vi "email.vi"(1 "Body":string="[No Body]", 2 "Enable":bool) -> ()   [LabVIEW 2011]
panel:
  in  "CC (Carbon Copy Recipient - Optional) 2":string
  out "error out":errorcluster
  in  "CC (Carbon Copy Recipient - Optional)":string
  in  "Attachment - Optional":path
  in  "Port":i32=587
  in  "Enable SSL":bool=TRUE
  in  "GMAIL Account Password":string="joblhzitaafwukgr"
  in  "GMAIL Account User ID":string="hvac.labview"
  in  "Outgoing Mail Server (SMTP)":string="smtp.gmail.com"
  in  "Subject":string="Automatic Email: HVAC Project"
  in  "Recipient's Name":string="HVAC Member"
  in  "Recipient's Email":string="kth.ee.hvac@gmail.com"
  in  "Sender's Name":string="hvac.labview"
  in  "Sender's Email":string="hvac.labview@gmail.com"
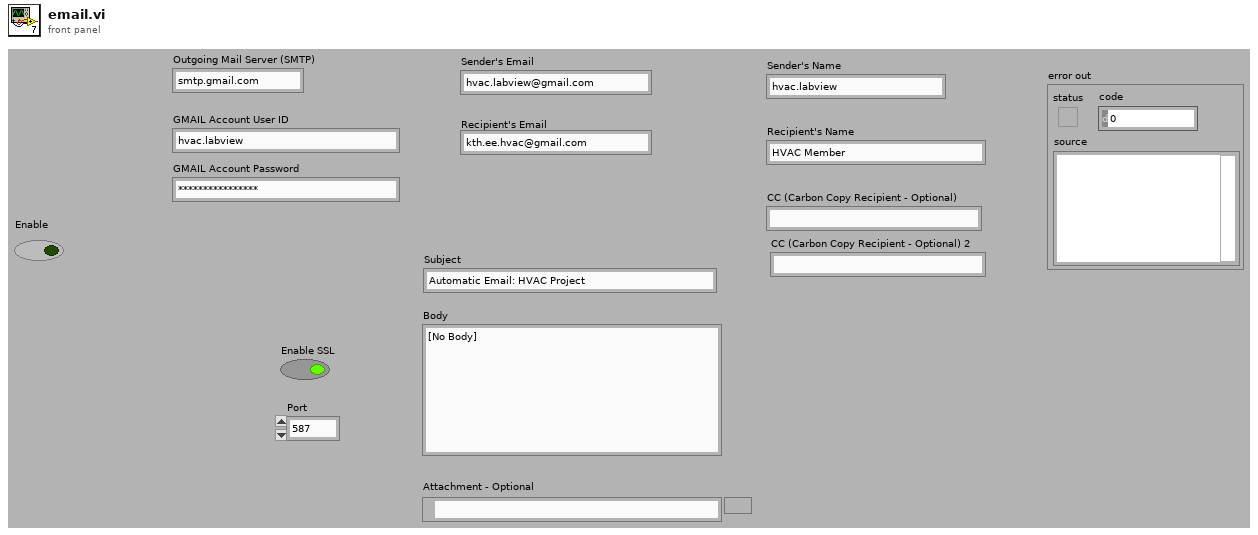
[diagram p1: front panel]
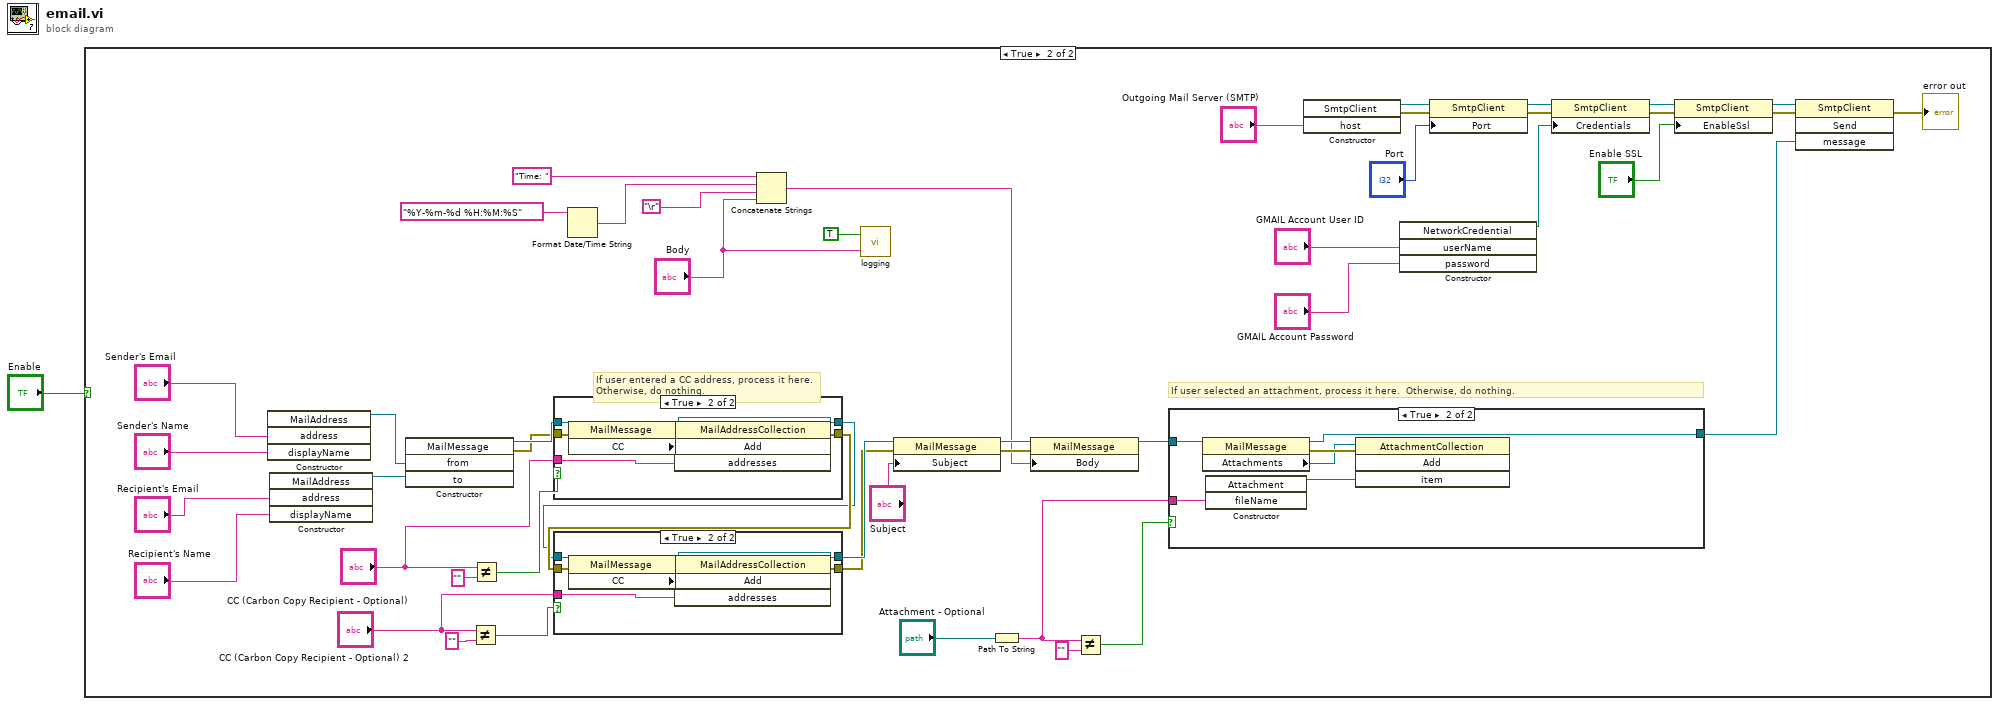
[diagram p0: block diagram]
diagram:
  n1 = case shown="True" "Enable" {
    frame False {
    }
    frame True {
      # "If user selected an attachment, process it here.  Otherwise, do nothing."
      # "If user entered a CC address, process it here.\nOtherwise, do nothing."
      n2 = constructor class="MailAddress"("address"="Sender's Email", "displayName"="Sender's Name") -> (reference out=w49:refnum<k24>)  [unwired: 3 in, 4 out]
      n3 = constructor class="MailAddress"("address"="Recipient's Email", "displayName"="Recipient's Name") -> (reference out=w50:refnum<k24>)  [unwired: 3 in, 4 out]
      n4 = constructor class="MailMessage"("from"=w49, "to"=w50) -> (reference out=w18:refnum<k24>, error out=w17:errorcluster)  [unwired: 3 in, 3 out]
      n5 = Not Equal?(x="CC (Carbon Copy Recipient - Optional) 2", y="") -> (x != y?=w7:bool)
      n6 = Not Equal?(x="CC (Carbon Copy Recipient - Optional)", y="") -> (x != y?=w20:bool)
      n7 = case shown="True" w20 {
        tunnel: "CC (Carbon Copy Recipient - Optional)" -> [_ w66]
        tunnel: w18 -> [w61 w65]
        tunnel: w17 -> [w60 w64]
        tunnel: [w61 w63] -> w5
        tunnel: [w60 w62] -> w6
        frame False {
        }
        frame True {
          n8 = property class="MailMessage"(reference=w65, error in=w64) -> (reference out=w63:refnum<k24>, error out=w68:errorcluster, "CC"=w67:refnum<k24>)
          n9 = invoke class="MailAddressCollection" method="Add"(reference=w67, error in=w68, "addresses"=w66) -> (error out=w62:errorcluster)  [unwired: 1 in, 3 out]
        }
      }
      n10 = case shown="True" w7 {
        tunnel: "CC (Carbon Copy Recipient - Optional) 2" -> [_ w57]
        tunnel: w5 -> [w52 w56]
        tunnel: w6 -> [w51 w55]
        tunnel: [w52 w54] -> w3
        tunnel: [w51 w53] -> w2
        frame False {
        }
        frame True {
          n11 = property class="MailMessage"(reference=w56, error in=w55) -> (reference out=w54:refnum<k24>, error out=w59:errorcluster, "CC"=w58:refnum<k24>)
          n12 = invoke class="MailAddressCollection" method="Add"(reference=w58, error in=w59, "addresses"=w57) -> (error out=w53:errorcluster)  [unwired: 1 in, 3 out]
        }
      }
      n13 = Format Date/Time String(time format string (%c)="%Y-%m-%d %H:%M:%S") -> (date/time string=w12:string)  [unwired: 2 in]
      n14 = Concatenate Strings("Time: ", w12, "\r", "Body") -> (w10:string)
      n15 = call "logging.vi"("data"="Body", "Boolean"=TRUE) -> ()  [unwired: 1 in]
      n16 = property class="MailMessage"(reference=w3, error in=w2, "Subject"="Subject") -> (reference out=w41:refnum<k24>, error out=w48:errorcluster)
      n17 = Path To String(path="Attachment - Optional") -> (string=w22:string)
      n18 = property class="MailMessage"(reference=w41, error in=w48, "Body"=w10) -> (reference out=w27:refnum<k24>)  [unwired: 1 out]
      n19 = Not Equal?(x=w22, y="") -> (x != y?=w23:bool)
      n20 = case shown="True" w23 {
        tunnel: w27 -> [w69 w72]
        tunnel: [w69 w71] -> w26
        tunnel: w22 -> [_ w70]
        frame False {
        }
        frame True {
          n21 = property class="MailMessage"(reference=w72) -> (reference out=w71:refnum<k24>, error out=w75:errorcluster, "Attachments"=w73:refnum<k24>)  [unwired: 1 in]
          n22 = constructor class="Attachment"("fileName"=w70) -> (reference out=w74:refnum<k24>)  [unwired: 3 in, 3 out]
          n23 = invoke class="AttachmentCollection" method="Add"(reference=w73, error in=w75, "item"=w74) -> ()  [unwired: 1 in, 4 out]
        }
      }
      n24 = constructor class="SmtpClient"("host"="Outgoing Mail Server (SMTP)") -> (reference out=w35:refnum<k24>, error out=w31:errorcluster)  [unwired: 3 in, 2 out]
      n25 = constructor class="NetworkCredential"("userName"="GMAIL Account User ID", "password"="GMAIL Account Password") -> (reference out=w36:refnum<k24>)  [unwired: 3 in, 4 out]
      n26 = property class="SmtpClient"(reference=w35, error in=w31, "Port"="Port") -> (reference out=w34:refnum<k24>, error out=w30:errorcluster)
      n27 = property class="SmtpClient"(reference=w34, error in=w30, "Credentials"=w36) -> (reference out=w33:refnum<k24>, error out=w29:errorcluster)
      n28 = property class="SmtpClient"(reference=w33, error in=w29, "EnableSsl"="Enable SSL") -> (reference out=w32:refnum<k24>, error out=w28:errorcluster)
      n29 = invoke class="SmtpClient" method="Send"(reference=w32, error in=w28, "message"=w26) -> (error out=→"error out":errorcluster)  [unwired: 1 in, 3 out]
    }
  }
